vi "Joystick Manipulator.vi"() -> (0 "Secondary Controller":T1)   [LabVIEW 2014]
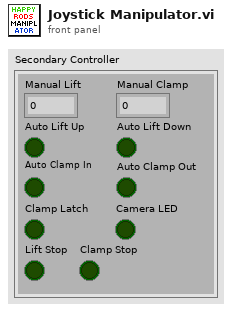
[diagram p1: front panel]
types:
  T1 = cluster{"Manual Lift":dbl, "Manual Clamp":dbl, "Auto Lift Up":bool, "Auto Lift Down":bool, "Auto Clamp In":bool, "Auto Clamp Out":bool, "Clamp Latch":bool, "Camera LED":bool, "Lift Stop":bool, "Clamp Stop":bool}
  T2 = cluster{"Buttons":cluster{"1":bool, "2":bool, "3":bool, "4":bool, "5":bool, "6":bool, "7":bool, "8":bool, "9":bool, "10":bool}, "Axes":cluster{"X":dbl, "Y":dbl, "Throttle":dbl}}
  T3 = cluster{"Y":dbl, "X":dbl, "3":bool, "2":bool, "4":bool, "5":bool, "1":bool, "10":bool, "6":bool, "7":bool}
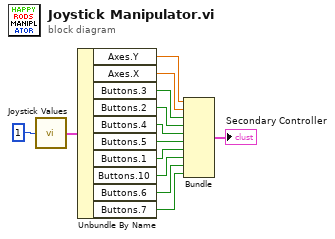
[diagram p0: block diagram]
diagram:
  n1 = call "Joystick Values.vi"("Joystick Index"=1) -> ("Joystick"=w12:T2)
  n2 = Unbundle By Name(w12) -> ("Axes.Y"=w11:dbl, "Axes.X"=w10:dbl, "Buttons.3"=w9:bool, "Buttons.2"=w8:bool, "Buttons.4"=w7:bool, "Buttons.5"=w6:bool, "Buttons.1"=w5:bool, "Buttons.10"=w4:bool, "Buttons.6"=w3:bool, "Buttons.7"=w2:bool)
  n3 = Bundle("Y"=w11, "X"=w10, "3"=w9, "2"=w8, "4"=w7, "5"=w6, "1"=w5, "10"=w4, "6"=w3, "7"=w2) -> (→"Secondary Controller":T3)  [unwired: 1 in]
